vi "Global 3.vi"() -> ()   [LabVIEW 2022 SP3]
panel:
  in  "Abort":bool
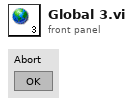
[diagram p1: front panel]
diagram:
